vi "close.vi"(8 "error in (no error)":errorcluster, 11 "Simple Sequencer API in":refnum<class "Simple Sequencer API.lvclass">) -> (0 "error out":errorcluster, 3 "Simple Sequencer API out":refnum<class "Simple Sequencer API.lvclass">)   [LabVIEW 2014, in "Simple Sequencer API.lvclass"]
doc: "Unitializes and destroys the session."
uses:
  Simple Sequencer API.lvclass
  Simple Sequencer API.lvclass/Simple Sequencer API.ctl
  module/execution/Simple Sequencer TBM runtime.lvclass
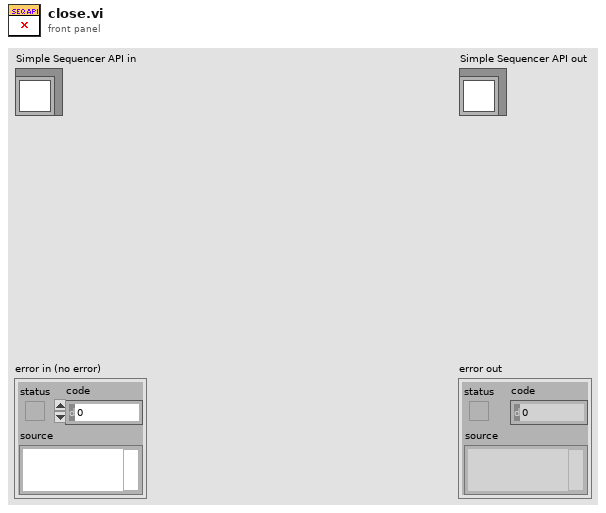
[diagram p1: front panel]
types:
  T1 = typedef "AMC.lvlib/Message Queue.ctl" = refnum<queue>
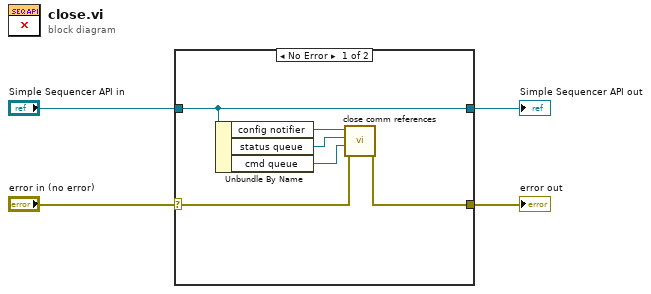
[diagram p0: block diagram]
diagram:
  n1 = case shown="No Error" "error in (no error)" {
    selector: "error in (no error)" -> [w6 w12]
    tunnel: [w5 w12] -> w3
    tunnel: [w10 w11] -> w1
    tunnel: "Simple Sequencer API in" -> [w10 w11]
    frame No Error {
      n2 = Unbundle By Name(w10) -> ("config notifier"=w9:refnum<notifier>, "status queue"=w8:T1, "cmd queue"=w7:T1)
      n3 = call "close comm references.vi"("error in (no error)"=w6, "status queue"=w7, "cmd queue"=w8, "configuration notifier"=w9) -> ("error out"=w5:errorcluster)  [unwired: 7 in]
    }
    frame Error {
    }
  }
  "error out" <- w3
  "Simple Sequencer API out" <- w1
